vi "local_variable.vi"() -> ()   [LabVIEW 2014]
panel:
  in  "Knob":i32(knob) scale=0.0..10.0
  in  "stop":bool
  out "Boolean 2":bool
  out "Boolean":bool
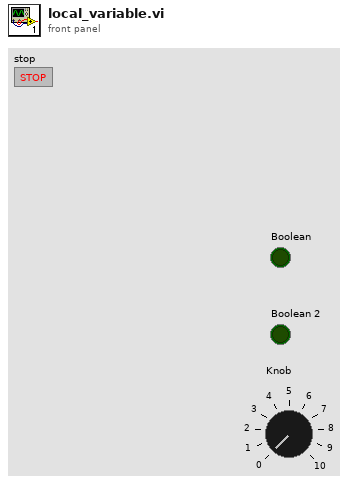
[diagram p1: front panel]
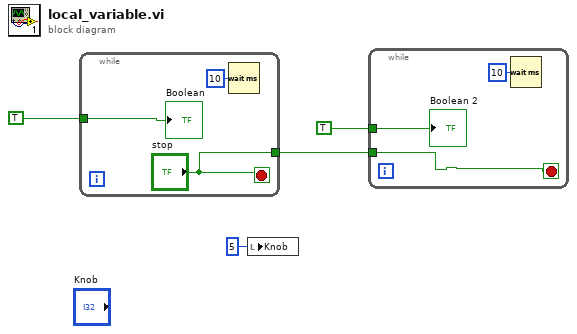
[diagram p0: block diagram]
diagram:
  n1 = while {
    tunnel: TRUE ("Boolean") -> [w7]
    tunnel: ["stop"] -> w2
    stop <- "stop" stop-if-true
    n2 = Wait (ms)(milliseconds to wait=u32 10) -> ()  [unwired: 1 out]
    "Boolean" <- w7
  }
  n3 = local write "Knob"(5 ("Knob")) -> ()
  n4 = while {
    tunnel: TRUE ("Boolean 2") -> [w10]
    tunnel: w2 -> [w8]
    stop <- w8 stop-if-true
    n5 = Wait (ms)(milliseconds to wait=u32 10) -> ()  [unwired: 1 out]
    "Boolean 2" <- w10
  }
